vi "AI Asynchronous Timing and Sync.vi"(4 "Status Notifier":refnum<notifier>, 6 "Initialization Status Notifier":refnum<notifier>, 7 "Device Clock":string, 9 "Inputs FIFO":refnum<k33>, 10 "Outputs FIFO":refnum<k33>, 11 "Device Ref":T1 format="%.0x") -> ()   [LabVIEW 2013]
uses:
  <vilib>/K2Labs/HiLab API/Custom Device API/Controls/Custom Device Item Reference.ctl
  <vilib>/K2Labs/HiLab API/Custom Device API/Controls/Custom Device Channel Type.ctl
  <vilib>/Platform/TimedLoop/XDataNode/timing_clust.ctl
  <vilib>/Platform/TimedLoop/XDataNode/nitl_modes.ctl
  <vilib>/Platform/TimedLoop/XDataNode/wakeup.ctl
  <vilib>/DAQmx/read.llb/DAQmx Read (Analog 1D DBL NChan 1Samp).vi
  <vilib>/DAQmx/miscellaneous.llb/DAQmx Fill In Error Info.vi
  <vilib>/Platform/TimedLoop/XDataNode/XDataNode.xnode
  <vilib>/K2Labs/HiLab API/Custom Device API/Custom Device API Library.lvlib
  <vilib>/Platform/TimedLoop/XDataNode/XDNodeRunTimeDep.lvlib
  <vilib>/DAQmx/configure/timing.llb/DAQmx Timing (Sample Clock).vi
panel:
  out "error out":errorcluster
  # "Do not delete!"
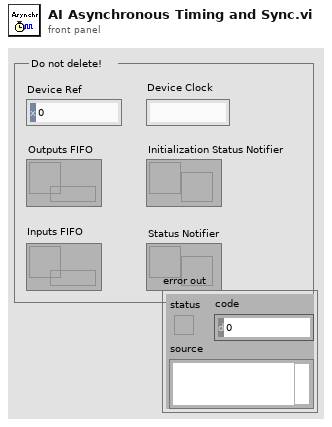
[diagram p1: front panel]
types:
  T1 = typedef "Custom Device API Library.lvlib/Custom Device Item Reference.ctl" = u64
  T2 = typedef "Custom Device API Library.lvlib/Custom Device Channel Type.ctl" = enum16{"Input", "Output"}
  T3 = typedef "AI Device Settings.ctl" = cluster{"Dev":string, "task":refnum<k21>, "Indexs":i32[], "Scales":T4[]}
  T4 = typedef "AI Scale.ctl" = cluster{"Factor":dbl, "Offset":dbl}
  T5 = typedef "XDNodeRunTimeDep.lvlib/timing_clust.ctl" = cluster{"Expected End [f-1]":u64, "Actual End [f-1]":u64, "Finished Late? [f-1]":bool, "Expected End [i-1]":u64, "Actual End [i-1]":u64, "Finished Late? [i-1]":bool, "Expected Start [i]":u64, "Actual Start [i]":u64, "Expected Start [f]":u64, "Actual Start [f]":u64, "Source Name":string, "Structure Name":string, "Period":i64, "Deadline":i64, "Offset":i64, "Start":i64, "Priority":i32, "Timeout":i32, "Mode":T6, "Wakeup Reason":T7, "Error":errorcluster, "Source Type":string, "Secondary Source Type":string, "Global End Time":u64, "Global Start Time":u64, "Frame Duration":u64, "Iteration Duration":u64, "Assigned CPU":i32, "I/O Scan Engine Mode":u32}
  T6 = typedef "XDNodeRunTimeDep.lvlib/nitl_modes.ctl" = enum32{"No Change", "Process missed periods, maintain original phase", "Discard missed periods, maintain original phase", "Process missed periods, ignore original phase", "Discard missed periods, ignore original phase"}
  T7 = typedef "XDNodeRunTimeDep.lvlib/wakeup.ctl" = enum32{"Normal", "Aborted", "Asynchronous wakeup", "Timing source error", "Timed loop error", "Timeout"}
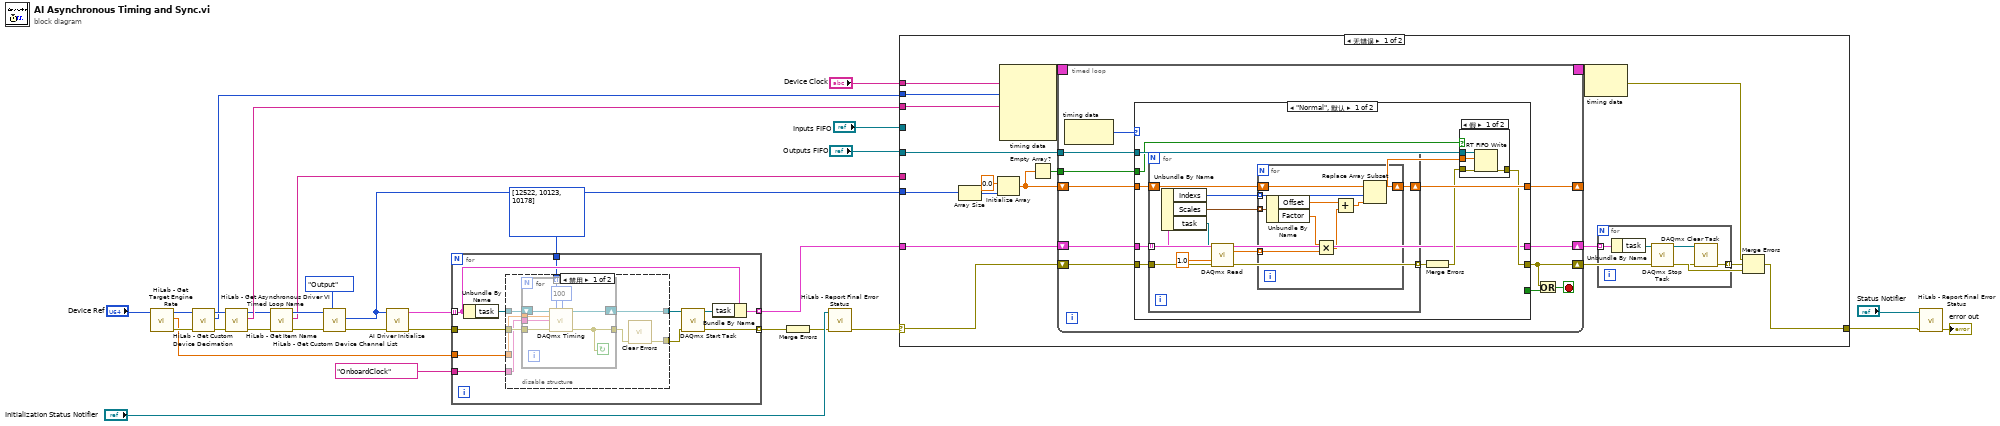
[diagram p0: block diagram]
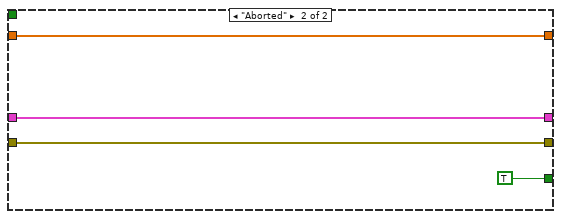
[diagram p4: hidden frame]
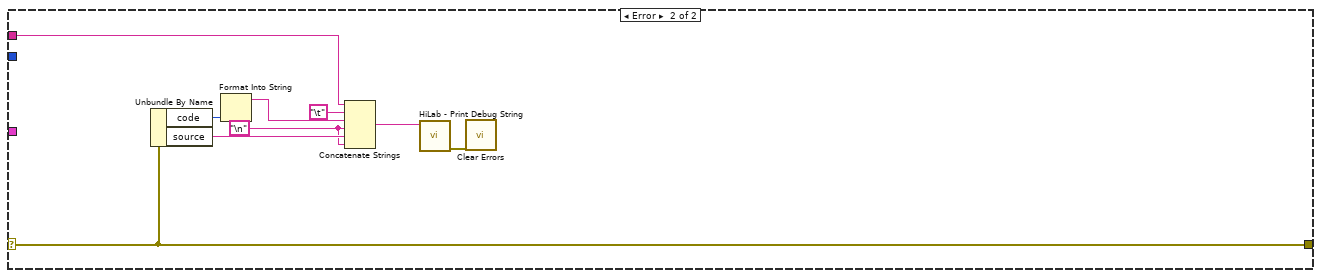
[diagram p5: hidden frame]
diagram:
  w1 = i32[] [12522, 10123, 10178] items=["有限采样"=10178, "连续采样"=10123, "硬件定时单点"=12522]
  n1 = call <vilib>:"HiLab - Get Target Engine Rate.vi"("Item Ref in"="Device Ref") -> ("error out"=w4:errorcluster, "Rate(Hz)"=w3:dbl, "Item Ref out"=w5:T1)  [unwired: 7 in, 1 out]
  n2 = call <vilib>:"HiLab - Get Custom Device Decimation.vi"("error in (no error)"=w4, "Device Ref in"=w5) -> ("error out"=w21:errorcluster, "Decimation"=w20:i32, "Device Ref out"=w22:T1)  [unwired: 7 in]
  n3 = call <vilib>:"HiLab - Get Asynchronous Driver VI Timed Loop Name.vi"("error in (no error)"=w21, "Device Ref in"=w22) -> ("error out"=w18:errorcluster, "Timed Loop Name"=w24:string, "Device Ref out"=w19:T1)  [unwired: 7 in]
  n4 = call <vilib>:"HiLab - Get Item Name.vi"("error in (no error)"=w18, "Item Ref in"=w19) -> ("error out"=w15:errorcluster, "Name"=w16:string, "Item Ref out"=w17:T1)  [unwired: 6 in, 1 out]
  n5 = call <vilib>:"HiLab - Get Custom Device Channel List.vi"("Type"=Custom_Device_Channel_Type."Output", "error in (no error)"=w15, "Device Ref in"=w17) -> ("error out"=w13:errorcluster, "Channel Refs"=w14:T1[])  [unwired: 6 in, 1 out]
  n6 = call "AI Driver Initialize.vi"("error in (no error)"=w13, "Channel Refs"=w14) -> ("error out"=w11:errorcluster, "Tasks"=w12:T3[])  [unwired: 8 in]
  n7 = for {
    tunnel: w12 -> [w42] mode=indexing
    tunnel: w11 -> [w37]
    tunnel: [w40] -> w10 mode=indexing
    tunnel: [w39] -> w8 mode=indexing
    tunnel: w3 -> [w34]
    tunnel: tag "OnboardClock" ("采样时钟源") -> [w33]
    tunnel: w1 -> [w32]
    n8 = Unbundle By Name(w42) -> ("task"=w38:refnum<k21>)
    n9 = disable-structure shown="禁用" {
      disable-tunnel: w38 -> [w50 w60]
      disable-tunnel: w37 -> [w49 w59]
      disable-tunnel: [w47 w60] -> w36
      disable-tunnel: [w46 w59] -> w35
      disable-tunnel: w34 -> [w45 _]
      disable-tunnel: w33 -> [w44 _]
      disable-tunnel: w32 -> [w43 _]
      frame Disabled {
        n10 = for {
          tunnel: w49 -> [w57]
          tunnel: [w51] -> w48
          tunnel: w45 -> [w54]
          tunnel: w44 -> [w53]
          shift-right: [w56] -> w47
          shift-left: w50 -> [w58]
          tunnel: w43 -> [w52] mode=indexing
          stop <- w51 continue-if-true
          n11 = call-poly <vilib>:"DAQmx Timing.vi"("task/channels in"=w58, "sample mode"=w52, "samples per channel"=100, "rate"=w54, "source"=w53, "error in"=w57) -> ("task out"=w56:refnum<k21>, "error out"=w51:errorcluster)  [unwired: 8 in]
        }
        n12 = call <vilib>:"Clear Errors.vi"("error in (no error)"=w48) -> ("error out"=w46:errorcluster)  [unwired: 6 in]
      }
      frame Enabled {
      }
    }
    n13 = call <vilib>:"DAQmx Start Task.vi"("task/channels in"=w36, "error in"=w35) -> ("task out"=w41:refnum<k21>, "error out"=w40:errorcluster)  [unwired: 12 in]
    n14 = Bundle By Name(cluster=w42, "task"=w41) -> (w39:T3)
  }
  n15 = Merge Errors(w10) -> (w9:errorcluster)
  n16 = call <vilib>:"HiLab - Report Final Error Status.vi"("error in (no error)"=w9, "Status Notifier"="Initialization Status Notifier") -> ("error out"=w7:errorcluster)  [unwired: 9 in]
  n17 = case shown="无错误" w7 {
    selector: w7 -> [w61 w150]
    tunnel: [w68 w150] -> w29
    tunnel: "Inputs FIFO" -> [_ _]
    tunnel: "Outputs FIFO" -> [w78 _]
    tunnel: w14 -> [w74 _]
    tunnel: w24 -> [w71 _]
    tunnel: "Device Clock" -> [w70 _]
    tunnel: w20 -> [w69 _]
    tunnel: w8 -> [w62 _]
    tunnel: w16 -> [_ w144]
    frame No Error {
      n18 = Array Size(array=w74) -> (size(s)=w75:i32)
      n19 = Initialize Array(0.0 ("元素"), w75) -> (w66:dbl[])
      n20 = node-c288(w70, w69, w71) -> (w73:T5)  [unwired: 2 in]
      n21 = Empty Array?(array=w66) -> (empty?=w77:bool)
      n22 = timed-loop {
        shift-right: [w92] -> w63
        shift-left: w61 -> [w94]
        tunnel: w78 -> [w90]
        shift-right: [w88] -> _
        shift-left: w66 -> [w89]
        tunnel: w77 -> [w87]
        timing: w73 -> [_]
        timing-out: [_] -> w72
        shift-right: [w84] -> w67
        shift-left: w62 -> [w85]
        stop <- w91 stop-if-true
        n23 = node-c288() -> (w86:T7)  [unwired: 1 in]
        n24 = case shown="\"Normal\", 默认" w86 {
          tunnel: w94 -> [w100 w133]
          tunnel: [w102 w133] -> w92
          tunnel: [_ TRUE] -> w93
          tunnel: w90 -> [w105 _]
          tunnel: w89 -> [w104 w132]
          tunnel: [w103 w132] -> w88
          tunnel: w87 -> [w101 _]
          tunnel: w85 -> [w97 w130]
          tunnel: [w97 w130] -> w84
          frame "Normal", Default {
            n25 = for {
              tunnel: w97 -> [w107] mode=indexing
              tunnel: w100 -> [w113]
              tunnel: [w112] -> w99 mode=indexing
              shift-right: [w114] -> w103
              shift-left: w104 -> [w115]
              n26 = Unbundle By Name(w107) -> ("Indexs"=w109:i32[], "Scales"=w106:T4[], "task"=w110:refnum<k21>)
              n27 = call-poly <vilib>:"DAQmx Read.vi"("task/channels in"=w110, "timeout"=1.0, "error in"=w113) -> ("data"=w108:dbl[], "error out"=w112:errorcluster)  [unwired: 10 in, 1 out]
              n28 = for {
                shift-right: [w123] -> w114
                shift-left: w115 -> [w124]
                tunnel: w109 -> [w122] mode=indexing
                tunnel: w108 -> [w119] mode=indexing
                tunnel: w106 -> [w121] mode=indexing
                n29 = Unbundle By Name(w121) -> ("Offset"=w118:dbl, "Factor"=w120:dbl)
                n30 = Multiply(x=w120, y=w119) -> (x*y=w117:dbl)
                n31 = Add(x=w118, y=w117) -> (x+y=w116:dbl)
                n32 = Replace Array Subset(array=w124, new element=w116, index=w122) -> (w123:dbl[])
              }
            }
            n33 = Merge Errors(w99) -> (w98:errorcluster)
            n34 = case shown="假" w101 {
              tunnel: w105 -> [w128 _]
              tunnel: w103 -> [w127 _]
              tunnel: w98 -> [w126 w129]
              tunnel: [w125 w129] -> w102
              frame False {
                n35 = RT FIFO Write(0:w128, 1:w127, 3:w126) -> (11:w125:errorcluster)  [unwired: 2 in, 3 out]
              }
              frame True {
              }
            }
          }
          frame "Aborted" {
          }
        }
        n36 = Or(x=w92, y=w93) -> (x .or. y?=w91:bool)
      }
      n37 = node-c288(w72) -> (w65:errorcluster)
      n38 = for {
        tunnel: w67 -> [w83] mode=indexing
        tunnel: [w80] -> w64 mode=indexing
        n39 = Unbundle By Name(w83) -> ("task"=w79:refnum<k21>)
        n40 = call <vilib>:"DAQmx Stop Task.vi"("task/channels in"=w79) -> ("task out"=w82:refnum<k21>, "error out"=w81:errorcluster)  [unwired: 13 in]
        n41 = call <vilib>:"DAQmx Clear Task.vi"("task in"=w82, "error in"=w81) -> ("error out"=w80:errorcluster)  [unwired: 13 in]
      }
      n42 = Merge Errors(w65, w64, w63) -> (w68:errorcluster)
    }
    frame Error {
      w142 = "\n"
      n43 = Unbundle By Name(w150) -> ("code"=w149:i32, "source"=w147:string)
      n44 = Format Into String(w149) -> (resulting string=w148:string)  [unwired: 3 in, 1 out]
      n45 = Concatenate Strings(w144, "\t", w148, w142, w147, w142) -> (w146:string)
      n46 = call <vilib>:"HiLab - Print Debug String.vi"("Message"=w146) -> ("error out"=w145:errorcluster)  [unwired: 10 in]
      n47 = call <vilib>:"Clear Errors.vi"("error in (no error)"=w145) -> ()  [unwired: 6 in, 1 out]
    }
  }
  n48 = call <vilib>:"HiLab - Report Final Error Status.vi"("error in (no error)"=w29, "Status Notifier"="Status Notifier") -> ("error out"=→"error out":errorcluster)  [unwired: 9 in]
